vi "WriteInSharedVar.vi"() -> ()   [LabVIEW 2012]
panel:
  in  "refnum de variable partagée en entrée":refnum<k21>
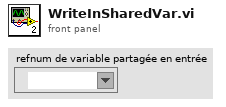
[diagram p1: front panel]
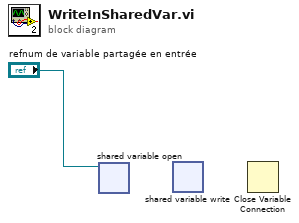
[diagram p0: block diagram]
diagram:
  n1 = shared-variable-open("refnum de variable partagée en entrée") -> ()  [unwired: 3 in, 2 out]
  n2 = shared-variable-write() -> ()  [unwired: 3 in, 2 out]
  n3 = Close Variable Connection() -> ()  [unwired: 2 in, 1 out]
